vi "get_date.vi"() -> (3 "日期/时间字符串":string)   [LabVIEW 2012]
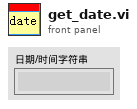
[diagram p1: front panel]
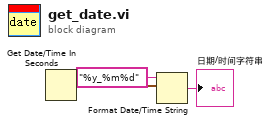
[diagram p0: block diagram]
diagram:
  n1 = Get Date/Time In Seconds() -> (seconds since 1Jan1904=w3:timestamp)
  n2 = Format Date/Time String(time format string (%c)="%y_%m%d" ("时间格式字符串(%c)"), seconds (now)=w3) -> (date/time string=→"日期/时间字符串":string)  [unwired: 1 in]
